vi "Run.vi"(8 "error in (no error)":errorcluster caption="entrée d'erreur (pas d'erreur)", 11 "Class Camera IV3-500CA en entrée":refnum<class "Class Camera IV3-500CA.lvclass">) -> (0 "error out":errorcluster caption="sortie d'erreur", 3 "Class Camera IV3-500CA en sortie":refnum<class "Class Camera IV3-500CA.lvclass">)   [LabVIEW 2020, in "Library Instrument & Equipement.lvlib" / "Library Camera.lvlib" / "Class Camera IV3-500CA.lvclass"]
uses:
  Class Camera IV3-500CA.lvclass
  C:/Users/ngarcin/OneDrive - Altyor/Standard TB/Class/Camera/Class Camera Pattern Matching (Default)/Class Pattern Matching (Default).lvclass
  Class Camera  IV3-500CA - Change Program/Class Camera  IV3-500CA - Change Program.lvclass
  Class Camera  IV3-500CA - Start Program/Class Camera  IV3-500CA - Start Program.lvclass
  Class Camera IV3-500CA.lvclass/Class Camera IV3-500CA.ctl
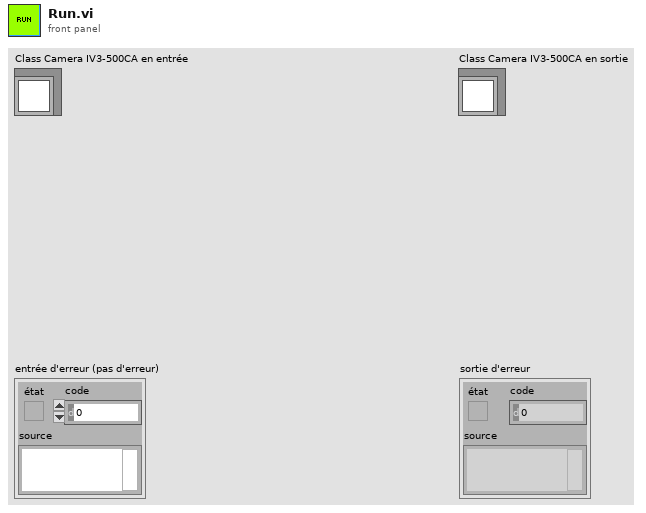
[diagram p1: front panel]
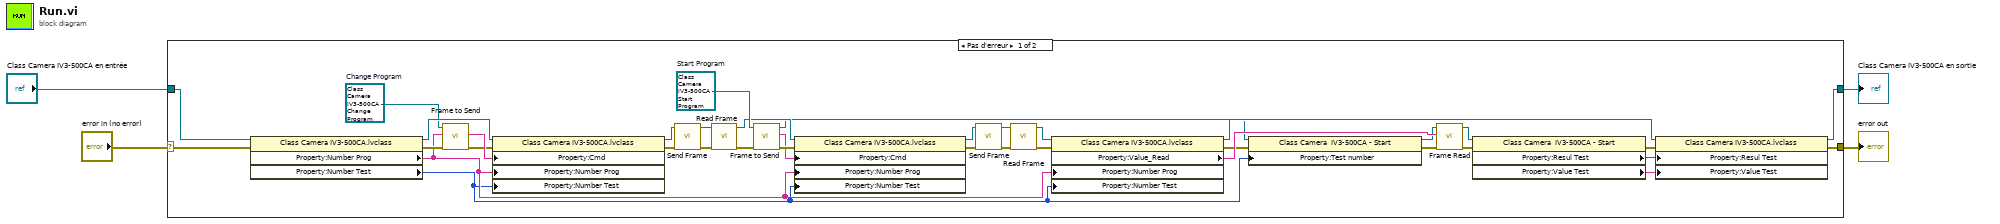
[diagram p0: block diagram]
diagram:
  n1 = case shown="Pas d'erreur" "error in (no error)" {
    selector: "error in (no error)" -> [w33 w43]
    tunnel: [w12 w43] -> w3
    tunnel: [w16 w42] -> w1
    tunnel: "Class Camera IV3-500CA en entrée" -> [w35 w42]
    frame No Error {
      w27 = refnum<class "Class Camera  IV3-500CA - Start Program.lvclass"> refnum  # Start Program
      w11 = refnum<class "Class Camera  IV3-500CA - Change Program.lvclass"> refnum  # Change Program
      n2 = property class="Class Camera IV3-500CA.lvclass"(reference=w35, error in=w33) -> (reference out=w34:refnum<class "Class Camera IV3-500CA.lvclass">, error out=w10:errorcluster, "Property:Number Prog"=w9:string, "Property:Number Test"=w7:u16)
      n3 = call-dynamic "Frame to Send.vi"("error in (no error)"=w10, "Number Prog"=w9, "Class Camera  IV3-500CA - Start Program en Entrée"=w11) -> ("error out"=w37:errorcluster, "Frame to Write"=w38:string)  [unwired: 6 in, 1 out]
      n4 = property class="Class Camera IV3-500CA.lvclass"(reference=w34, error in=w37, "Property:Cmd"=w38, "Property:Number Prog"=w9, "Property:Number Test"=w7) -> (reference out=w39:refnum<class "Class Camera IV3-500CA.lvclass">, error out=w36:errorcluster)
      n5 = call-dynamic "Send Frame.vi"("error in (no error)"=w36, "Class Camera IV3-500CA (Default) en Entrée"=w39) -> ("error out"=w40:errorcluster, "Class Camera IV3-500CA (Default) en Sortie"=w41:refnum<class "Class Camera IV3-500CA.lvclass">)  [unwired: 8 in]
      n6 = call-dynamic "Read Frame.vi"("error in (no error)"=w40, "Class Camera IV3-500CA (Default) en Entrée"=w41) -> ("error out"=w26:errorcluster, "Class Camera IV3-500CA (Default) en Sortie"=w24:refnum<class "Class Camera IV3-500CA.lvclass">)  [unwired: 8 in]
      n7 = call-dynamic "Frame to Send.vi"("error in (no error)"=w26, "Class Camera  IV3-500CA - Start Program en Entrée"=w27) -> ("error out"=w31:errorcluster, "Frame to write"=w30:string, "Class Camera  IV3-500CA - Start Program en Sortie"=w6:refnum<class "Class Camera  IV3-500CA - Start Program.lvclass">)  [unwired: 7 in]
      n8 = property class="Class Camera IV3-500CA.lvclass"(reference=w24, error in=w31, "Property:Cmd"=w30, "Property:Number Prog"=w9, "Property:Number Test"=w7) -> (reference out=w29:refnum<class "Class Camera IV3-500CA.lvclass">, error out=w32:errorcluster)
      n9 = call-dynamic "Send Frame.vi"("error in (no error)"=w32, "Class Camera IV3-500CA (Default) en Entrée"=w29) -> ("error out"=w28:errorcluster, "Class Camera IV3-500CA (Default) en Sortie"=w25:refnum<class "Class Camera IV3-500CA.lvclass">)  [unwired: 8 in]
      n10 = call-dynamic "Read Frame.vi"("error in (no error)"=w28, "Class Camera IV3-500CA (Default) en Entrée"=w25) -> ("error out"=w20:errorcluster, "Class Camera IV3-500CA (Default) en Sortie"=w23:refnum<class "Class Camera IV3-500CA.lvclass">)  [unwired: 8 in]
      n11 = property class="Class Camera IV3-500CA.lvclass"(reference=w23, error in=w20, "Property:Number Prog"=w9, "Property:Number Test"=w7) -> (reference out=w22:refnum<class "Class Camera IV3-500CA.lvclass">, error out=w19:errorcluster, "Property:Value_Read"=w21:string)
      n12 = property class="Class Camera  IV3-500CA - Start"(reference=w6, error in=w19, "Property:Test number"=w7) -> (reference out=w5:refnum<class "Class Camera  IV3-500CA - Start Program.lvclass">, error out=w8:errorcluster)
      n13 = call-dynamic "Frame Read.vi"("error in (no error)"=w8, "Frame Read"=w21, "Class Camera  IV3-500CA - Start Program en Entrée"=w5) -> ("error out"=w17:errorcluster, "Class Camera  IV3-500CA - Start Program en Sortie"=w18:refnum<class "Class Camera  IV3-500CA - Start Program.lvclass">)  [unwired: 7 in]
      n14 = property class="Class Camera  IV3-500CA - Start"(reference=w18, error in=w17) -> (error out=w13:errorcluster, "Property:Resul Test "=w15:bool, "Property:Value Test"=w14:string)  [unwired: 1 out]
      n15 = property class="Class Camera IV3-500CA.lvclass"(reference=w22, error in=w13, "Property:Resul Test "=w15, "Property:Value Test"=w14) -> (reference out=w16:refnum<class "Class Camera IV3-500CA.lvclass">, error out=w12:errorcluster)
    }
    frame Error {
    }
  }
  "error out" <- w3
  "Class Camera IV3-500CA en sortie" <- w1
